vi "Finish.vi"(8 "error in (no error)":errorcluster, 11 "Processing":refnum<class "Processing.lvclass">) -> ()   [LabVIEW 2020, in "HTTP Server.lvlib" / "Server.lvclass"]
uses:
  Server.lvclass
  Server.lvclass/Server.ctl
  RequestTraceLog/RequestTraceLog.lvclass
  lv-http-util/HTTP Utils/Request/Request.lvclass
  Session/Session.lvclass
  Processing/Processing.lvclass
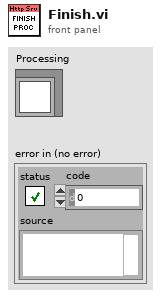
[diagram p1: front panel]
types:
  T1 = typedef "HTTP Server.lvlib/Session Debug Info.ctl" = cluster{"Loaded":bool, "Created":bool, "Destroyed":bool, "Created Time":timestamp}
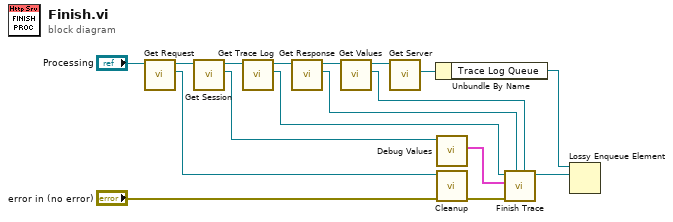
[diagram p0: block diagram]
diagram:
  n1 = call "Get Request.vi"("Processing in"="Processing") -> ("Request"=w2:refnum<class "Request.lvclass">, "Processing out"=w3:refnum<class "Processing.lvclass">)  [unwired: 9 in]
  n2 = call "Get Session.vi"("Processing in"=w3) -> ("Session"=w4:refnum<class "Session.lvclass">, "Processing out"=w5:refnum<class "Processing.lvclass">)  [unwired: 9 in]
  n3 = call "Get Trace Log.vi"("Processing in"=w5) -> ("Trace Log"=w6:refnum<class "RequestTraceLog.lvclass">, "Processing out"=w7:refnum<class "Processing.lvclass">)  [unwired: 9 in]
  n4 = call "Get Response.vi"("Processing in"=w7) -> ("Response"=w8:refnum<class "Response.lvclass">, "Processing out"=w9:refnum<class "Processing.lvclass">)  [unwired: 9 in]
  n5 = call "Get Values.vi"("Processing in"=w9) -> ("Values"=w10:refnum<class "Values.lvclass">, "Processing out"=w11:refnum<class "Processing.lvclass">)  [unwired: 9 in]
  n6 = call "Get Server.vi"("Processing in"=w11) -> ("Server"=w13:refnum<class "Server.lvclass">)  [unwired: 9 in, 1 out]
  n7 = Unbundle By Name(w13) -> ("Trace Log Queue"=w12:refnum<queue>)
  n8 = call "Debug Values.vi"("Session in"=w4) -> ("Session Debug Info"=w14:T1)  [unwired: 8 in, 2 out]
  n9 = call "Cleanup.vi"("error in (no error)"="error in (no error)", "Request in"=w2) -> ("error out"=w15:errorcluster)  [unwired: 9 in]
  n10 = call "Finish Trace.vi"("Values"=w10, "Response"=w8, "error in (no error)"=w15, "Session Debug Info"=w14, "RequestTraceLog in"=w6) -> ("RequestTraceLog out"=w17:refnum<class "RequestTraceLog.lvclass">)  [unwired: 5 in, 1 out]
  n11 = Lossy Enqueue Element(queue=w12, element=w17) -> ()  [unwired: 1 in, 4 out]
